vi "datapadding.vi"() -> ()   [LabVIEW 2020]
uses:
  common/record_file_handler/VFH-file_cluster-r140.ctl
  common/record_file_handler/VFH-file_cluster-NanoVNA.ctl
  common/record_file_handler/VFH-VNA_File_Handler.lvlib
panel:
  out "XY Graph":T1(graph)
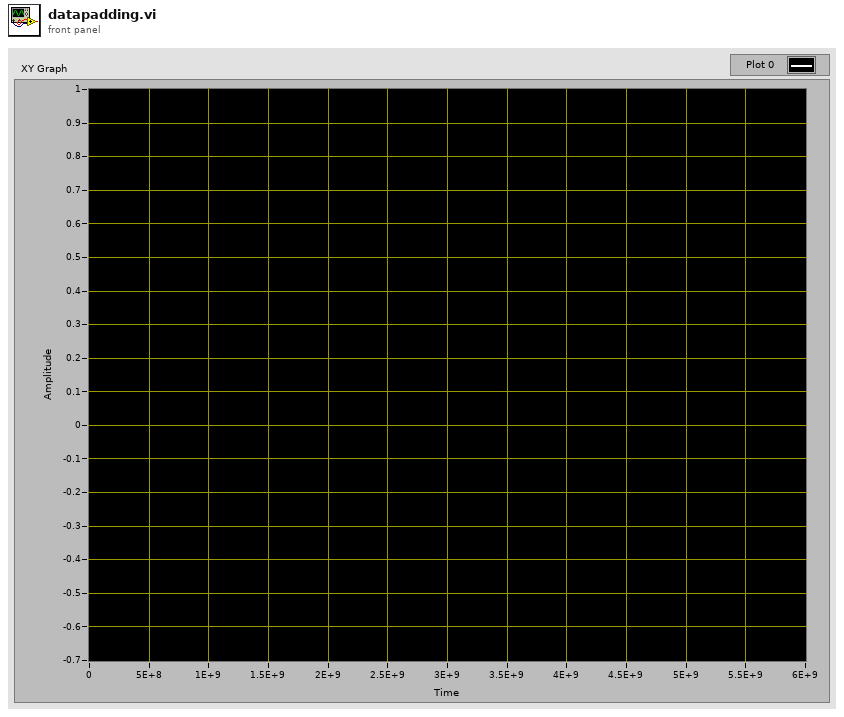
[diagram p1: front panel]
types:
  T1 = cluster{"Frequency":dbl[], "Reflection R":dbl[]}[]
  T2 = typedef "VFH-VNA_File_Handler.lvlib/VFH-file_cluster-NanoVNA.ctl" = cluster{"Frequency":dbl[], "S11_Real":dbl[], "S11_Imag":dbl[], "S21_Real":dbl[], "S21_Imag":dbl[], "S12_Real":dbl[], "S12_Imag":dbl[], "S22_Real":dbl[], "S22_Imag":dbl[]}
  T3 = typedef "VFH-VNA_File_Handler.lvlib/VFH-file_cluster-r140.ctl" = cluster{"Frequency":dbl[], "Permativity'":dbl[], "Permativity''":dbl[], "Q [S/m]":dbl[], "Tan":dbl[], "Reflection R":dbl[], "Reflection I":dbl[]}
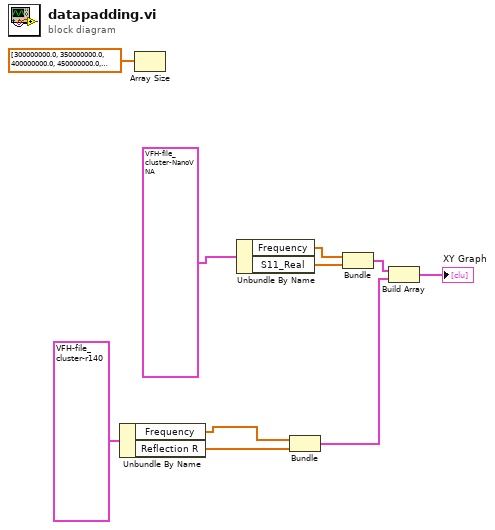
[diagram p0: block diagram]
diagram:
  n1 = Unbundle By Name(T3 {"Frequency"=[300000000.0, 350000000.0, 400000000.0, 450000000.0, 500000000.0, 550000000.0, 600000000.0, 650000000.0, 700000000.0, 750000000.0, 800000000.0, 850000000.0, 900000000.0, 950000000.0, 1000000000.0, 1050000000.0, 1100000000.0, 1150000000.0, 1200000000.0, 1250000000.0, 1300000000.0, 1350000000.0, 1400000000.0, 1450000000.0, 1500000000.0, 1550000000.0, 1600000000.0, 1650000000.0, 1700000000.0, 1750000000.0, 1800000000.0, 1850000000.0, 1900000000.0, 1950000000.0, 2000000000.0, 2050000000.0, 2100000000.0, 2150000000.0, 2200000000.0, 2250000000.0, 2300000000.0, 2350000000.0, 2400000000.0, 2450000000.0, 2500000000.0, 2550000000.0, 2600000000.0, 2650000000.0, 2700000000.0, 2750000000.0, 2800000000.0, 2850000000.0, 2900000000.0, 2950000000.0, 3000000000.0, 3050000000.0, 3100000000.0, 3150000000.0, 3200000000.0, 3250000000.0, 3300000000.0, 3350000000.0, 3400000000.0, 3450000000.0, 3500000000.0, 3550000000.0, 3600000000.0, 3650000000.0, 3700000000.0, 3750000000.0, 3800000000.0, 3850000000.0, 3900000000.0, 3950000000.0, 4000000000.0, 4050000000.0, 4100000000.0, 4150000000.0, 4200000000.0, 4250000000.0, 4300000000.0, 4350000000.0, 4400000000.0, 4450000000.0, 4500000000.0, 4550000000.0, 4600000000.0, 4650000000.0, 4700000000.0, 4750000000.0, 4800000000.0, 4850000000.0, 4900000000.0, 4950000000.0, 5000000000.0, 5050000000.0, 5100000000.0, 5150000000.0, 5200000000.0, 5250000000.0, 5300000000.0, 5350000000.0, 5400000000.0, 5450000000.0, 5500000000.0, 5550000000.0, 5600000000.0, 5650000000.0, 5700000000.0, 5750000000.0, 5800000000.0, 5850000000.0, 5900000000.0, 5950000000.0], "Permativity'"=[79.07108000000001, 79.07034, 79.06462, 79.056, 79.04534, 79.03753999999999, 79.0347, 79.03193999999999, 79.02342, 79.01277999999999, 78.99972, 78.98438, 78.97855999999999, 78.97154, 78.96216, 78.9497, 78.93456, 78.91888, 78.90404, 78.89126000000002, 78.8751, 78.86262, 78.84502, 78.82257999999999, 78.80032000000001, 78.7757, 78.74557999999999, 78.71386, 78.68402, 78.6533, 78.6191, 78.57827999999999, 78.52912, 78.46958, 78.41691999999999, 78.37318, 78.33406, 78.29446, 78.24640000000002, 78.19012000000001, 78.1309, 78.07466, 78.0258, 77.97828, 77.92783999999999, 77.869, 77.80196, 77.72826, 77.64728, 77.56294, 77.47844, 77.39797999999999, 77.31918, 77.24488, 77.17128, 77.09276, 77.01019999999998, 76.92546, 76.83918, 76.75408, 76.67336, 76.59342000000001, 76.51224, 76.42232, 76.33938, 76.2553, 76.16848, 76.07957999999999, 75.9925, 75.90732, 75.82844000000001, 75.75160000000001, 75.67374, 75.59042, 75.50016, 75.40386, 75.33228000000001, 75.23586, 75.12482, 75.01174, 74.90554, 74.8112, 74.72470000000001, 74.64645999999999, 74.56688, 74.5045, 74.42942000000001, 74.3682, 74.296, 74.22968, 74.18003999999999, 74.13322, 74.08314, 74.03887999999999, 73.97104, 73.89056, 73.81594, 73.72461999999999, 73.63058000000001, 73.54686, 73.47466, 73.40158, 73.33064, 73.27372, 73.20532, 73.13356, 73.09074, 73.00046, 72.8972, 72.78979999999999, 72.66766, 72.52906, 72.39554, 72.24091999999999], "Permativity''"=[1.6255039999999998, 1.868498, 2.0571159999999997, 2.2177439999999997, 2.3622919999999996, 2.5154699999999997, 2.6785360000000003, 2.850908, 3.044002, 3.243128, 3.4423440000000007, 3.6347099999999997, 3.8279579999999997, 4.024862000000001, 4.228188, 4.43362, 4.6342099999999995, 4.833124, 5.032642, 5.228612, 5.425520000000001, 5.623486, 5.823044, 6.021953999999999, 6.221154, 6.421606, 6.621852, 6.820505999999999, 7.0202860000000005, 7.221314, 7.42462, 7.6280019999999995, 7.8291319999999995, 8.02201, 8.215602, 8.411694, 8.611638000000001, 8.815472, 9.024792000000001, 9.23303, 9.438149999999998, 9.639506, 9.840016, 10.03886, 10.23822, 10.434259999999998, 10.62636, 10.81722, 11.011700000000001, 11.2103, 11.4122, 11.61576, 11.8175, 12.01362, 12.20212, 12.38604, 12.5691, 12.75498, 12.94442, 13.139000000000001, 13.33632, 13.52916, 13.71348, 13.88894, 14.062120000000002, 14.234300000000001, 14.409719999999998, 14.591159999999999, 14.775060000000002, 14.95574, 15.13636, 15.31298, 15.483160000000002, 15.6504, 15.81628, 15.981440000000001, 16.15642, 16.31804, 16.49034, 16.66446, 16.83074, 16.998400000000004, 17.1663, 17.32796, 17.47976, 17.64352, 17.805699999999998, 17.96982, 18.14518, 18.325300000000002, 18.499299999999998, 18.66046, 18.810859999999998, 18.94634, 19.081899999999997, 19.23704, 19.3982, 19.56258, 19.7285, 19.88428, 20.03192, 20.171139999999998, 20.296879999999998, 20.41714, 20.542180000000002, 20.663259999999998, 20.793979999999998, 20.938679999999998, 21.11282, 21.30238, 21.50122, 21.70846, 21.908160000000002, 22.099800000000005], "Q [S/m]"=[0.0271287, 0.03638146, 0.04577604, 0.05551923999999999, 0.06570876, 0.0769664, 0.08940635999999999, 0.10308999999999999, 0.11853899999999999, 0.1353148, 0.1532018, 0.1718732, 0.19165880000000002, 0.2127132, 0.2352194, 0.2589806, 0.2835878, 0.309204, 0.33596719999999997, 0.3635932, 0.3923774, 0.42233660000000006, 0.453521, 0.4857634, 0.5191366, 0.5537258, 0.589412, 0.6260655999999999, 0.6639314, 0.7030296, 0.7434744, 0.7850581999999999, 0.8275355999999998, 0.8702363999999999, 0.9140898, 0.9593052, 1.0060600000000002, 1.0543980000000002, 1.1045340000000003, 1.155704, 1.20763, 1.260208, 1.313792, 1.3682640000000001, 1.423912, 1.480208, 1.537014, 1.594708, 1.6540120000000003, 1.7150199999999998, 1.7776560000000003, 1.8416700000000001, 1.906532, 1.971584, 2.036464, 2.101606, 2.1676279999999997, 2.235168, 2.3043620000000002, 2.375554, 2.4483279999999996, 2.521362, 2.593852, 2.665678, 2.738024, 2.811148, 2.885876, 2.9628000000000005, 3.0412399999999997, 3.1200300000000003, 3.199818, 3.2797460000000003, 3.359253999999999, 3.439074, 3.5195260000000004, 3.6007279999999993, 3.685092, 3.767344, 3.8529919999999995, 3.94003, 4.026156, 4.113552, 4.201936, 4.289698, 4.375902, 4.465972, 4.556546, 4.648526, 4.744376000000001, 4.842433999999999, 4.9398800000000005, 5.034816, 5.127714, 5.21735, 5.3077559999999995, 5.404424000000001, 5.503655999999999, 5.60471, 5.707116, 5.807495999999999, 5.906328, 6.003494, 6.097367999999999, 6.19029, 6.285334, 6.379862, 6.478058, 6.581386, 6.694846, 6.814214, 6.937613999999999, 7.06486, 7.190802, 7.315175999999999], "Tan"=[0.0205575, 0.02363082, 0.02601812, 0.028052840000000002, 0.029885299999999997, 0.03182628, 0.03389066, 0.03607288, 0.03852024, 0.04104564, 0.04357414, 0.04601808, 0.048468300000000006, 0.05096598, 0.05354698, 0.05615753999999999, 0.058709500000000005, 0.061241659999999996, 0.0637818, 0.06627618, 0.0687862, 0.07130736, 0.07385428000000001, 0.0763989, 0.07894833999999999, 0.08151758, 0.08409177999999999, 0.08664936, 0.08922122, 0.09181196, 0.09443788, 0.0970752, 0.0996972, 0.1022308, 0.1047682, 0.1073288, 0.10993499999999998, 0.1125936, 0.11533820000000002, 0.1180844, 0.12079899999999999, 0.12346539999999999, 0.12611219999999998, 0.128739, 0.13138060000000001, 0.133998, 0.1365824, 0.13916699999999999, 0.1418172, 0.144532, 0.147295, 0.1500784, 0.1528406, 0.1555264, 0.15811780000000003, 0.16066419999999998, 0.1632134, 0.1658096, 0.168461, 0.17118319999999998, 0.17393679999999997, 0.1766362, 0.179232, 0.18173940000000002, 0.184205, 0.1866662, 0.1891822, 0.19178820000000002, 0.1944278, 0.19702619999999998, 0.1996136, 0.20214720000000003, 0.2046036, 0.2070418, 0.20948700000000003, 0.21194459999999998, 0.2144688, 0.21689180000000002, 0.2195058, 0.222158, 0.22469260000000002, 0.2272174, 0.2297276, 0.2321338, 0.2344172, 0.2368118, 0.23922919999999998, 0.24163259999999998, 0.24422859999999996, 0.24687260000000003, 0.2493842, 0.25171520000000003, 0.2539152, 0.25589699999999993, 0.25796420000000003, 0.26034520000000005, 0.2627916, 0.2653468, 0.267939, 0.27036239999999995, 0.272637, 0.2748058, 0.27678579999999997, 0.2786422, 0.2806106, 0.2825414, 0.2844954, 0.2868298, 0.2896246, 0.2926564, 0.2958842, 0.29930660000000003, 0.3026174, 0.3059182], "Reflection R"=[0.9563704, 0.9414002, 0.9247411999999999, 0.9059240000000001, 0.8855024, 0.8633542000000001, 0.8395902, 0.8143844000000001, 0.7883522000000001, 0.7609335999999999, 0.7324565999999999, 0.7032166000000001, 0.6739214, 0.6433788, 0.6123486, 0.5807945999999999, 0.5489086, 0.5175911999999999, 0.48633800000000005, 0.4556078, 0.4245774, 0.3932044, 0.3617632, 0.3310108, 0.30149380000000003, 0.2725546, 0.24442719999999998, 0.2156358, 0.18743959999999998, 0.1598338, 0.1335008, 0.1081772, 0.08306316, 0.05885234, 0.03523574, 0.01166094, -0.0112239, -0.03295492, -0.05388126, -0.07428524, -0.094318, -0.11344019999999999, -0.13217859999999998, -0.150481, -0.16820279999999999, -0.1856306, -0.20200420000000002, -0.21786219999999998, -0.23093919999999998, -0.2456136, -0.26064980000000004, -0.2747486, -0.288448, -0.3011898, -0.3128512, -0.324151, -0.3351994, -0.34643159999999995, -0.3575456, -0.36866319999999997, -0.3791824, -0.38919739999999997, -0.39882399999999996, -0.4075296, -0.41552039999999996, -0.42310299999999995, -0.43109340000000007, -0.43894420000000006, -0.4473358, -0.45564020000000005, -0.4632442, -0.4704846, -0.4770398, -0.4829552, -0.48858379999999996, -0.4945457999999999, -0.5007142, -0.5070786, -0.5129922, -0.5186019999999999, -0.5234748, -0.528023, -0.5318077999999999, -0.5361992000000001, -0.5410092000000001, -0.5462636000000001, -0.5514082, -0.5562567999999999, -0.5603596, -0.5636416, -0.5665338, -0.5734653999999999, -0.5766823999999999, -0.5790569999999999, -0.582066, -0.5858825999999999, -0.5894844, -0.5926942, -0.5958612000000001, -0.598381, -0.6025852, -0.6041282, -0.6085657999999999, -0.6097562, -0.6116034000000001, -0.614562, -0.6169844, -0.6190056, -0.6235666, -0.6252584, -0.6264618000000001, -0.6298440000000001, -0.630876, -0.6311298], "Reflection I"=[-0.2724698, -0.31527580000000005, -0.3569708, -0.39736259999999995, -0.43687820000000005, -0.47402820000000007, -0.5103186, -0.5448104, -0.577333, -0.6084758000000001, -0.6379132000000001, -0.6652576, -0.6909622000000001, -0.7150329999999999, -0.7374517999999999, -0.7579908, -0.7767417999999999, -0.7933899999999999, -0.8087218, -0.8230147999999999, -0.8356515999999999, -0.8470384, -0.8573310000000001, -0.8647012000000001, -0.8711336, -0.8764986, -0.8819204, -0.8860628, -0.8892678, -0.8904706000000001, -0.8907684, -0.8908866, -0.8899744, -0.8882756, -0.8864772000000001, -0.8838202000000001, -0.880477, -0.8765978000000001, -0.8724959999999999, -0.8680396, -0.8626924, -0.8571676, -0.8515086000000001, -0.8456258, -0.8394454, -0.8324263999999999, -0.8253484, -0.8182224, -0.8124207999999999, -0.8055906, -0.7983317999999999, -0.790975, -0.7835146, -0.7760478, -0.7686808, -0.7610172000000001, -0.7532197999999999, -0.745435, -0.7377613999999999, -0.7300576, -0.722393, -0.715164, -0.7083980000000001, -0.701418, -0.6942134, -0.686626, -0.6787333999999999, -0.6708944000000001, -0.6632136000000001, -0.6562418, -0.6494382, -0.6427252, -0.6360187999999999, -0.6294966, -0.6226278, -0.6150616000000001, -0.6078354, -0.6010314, -0.5946328000000001, -0.5886338, -0.582608, -0.5765022, -0.5701457999999999, -0.563566, -0.557402, -0.550292, -0.5437841999999999, -0.5379995999999999, -0.5325564, -0.5275712, -0.5224264, -0.5134958000000001, -0.5091794000000001, -0.5030577999999999, -0.49717399999999995, -0.4918436, -0.4859821999999999, -0.4802664, -0.4752636, -0.47164339999999993, -0.4649464, -0.46106559999999996, -0.4557778, -0.45077480000000003, -0.445472, -0.4396398, -0.4347174, -0.4301863999999999, -0.4259030000000001, -0.42265040000000004, -0.4174022, -0.411794, -0.40744800000000003, -0.40280940000000004]} ("Handled data")) -> ("Frequency"=w8:dbl[], "Reflection R"=w7:dbl[])
  n2 = Array Size(array=dbl[] [300000000.0, 350000000.0, 400000000.0, 450000000.0, 500000000.0, 550000000.0, 600000000.0, 650000000.0, 700000000.0, 750000000.0, 800000000.0, 850000000.0, 900000000.0, 950000000.0, 1000000000.0, 1050000000.0, 1100000000.0, 1150000000.0, 1200000000.0, 1250000000.0, 1300000000.0, 1350000000.0, 1400000000.0, 1450000000.0, 1500000000.0, 1550000000.0, 1600000000.0, 1650000000.0, 1700000000.0, 1750000000.0, 1800000000.0, 1850000000.0, 1900000000.0, 1950000000.0, 2000000000.0, 2050000000.0, 2100000000.0, 2150000000.0, 2200000000.0, 2250000000.0, 2300000000.0, 2350000000.0, 2400000000.0, 2450000000.0, 2500000000.0, 2550000000.0, 2600000000.0, 2650000000.0, 2700000000.0, 2750000000.0, 2800000000.0, 2850000000.0, 2900000000.0, 2950000000.0, 3000000000.0, 3050000000.0, 3100000000.0, 3150000000.0, 3200000000.0, 3250000000.0, 3300000000.0, 3350000000.0, 3400000000.0, 3450000000.0, 3500000000.0, 3550000000.0, 3600000000.0, 3650000000.0, 3700000000.0, 3750000000.0, 3800000000.0, 3850000000.0, 3900000000.0, 3950000000.0, 4000000000.0, 4050000000.0, 4100000000.0, 4150000000.0, 4200000000.0, 4250000000.0, 4300000000.0, 4350000000.0, 4400000000.0, 4450000000.0, 4500000000.0, 4550000000.0, 4600000000.0, 4650000000.0, 4700000000.0, 4750000000.0, 4800000000.0, 4850000000.0, 4900000000.0, 4950000000.0, 5000000000.0, 5050000000.0, 5100000000.0, 5150000000.0, 5200000000.0, 5250000000.0, 5300000000.0, 5350000000.0, 5400000000.0, 5450000000.0, 5500000000.0, 5550000000.0, 5600000000.0, 5650000000.0, 5700000000.0, 5750000000.0, 5800000000.0, 5850000000.0, 5900000000.0, 5950000000.0] ("Waveform Graph")) -> ()  [unwired: 1 out]
  n3 = Unbundle By Name(T2 {"Frequency"=array[801 elements], "S11_Real"=array[801 elements], "S11_Imag"=array[801 elements], "S21_Real"=array[801 elements], "S21_Imag"=array[801 elements], "S12_Real"=array[801 elements], "S12_Imag"=array[801 elements], "S22_Real"=array[801 elements], "S22_Imag"=array[801 elements]} ("avg output")) -> ("Frequency"=w5:dbl[], "S11_Real"=w4:dbl[])
  n4 = Bundle("Frequency"=w8, "Reflection R"=w7) -> (w2:cluster{"Frequency":dbl[], "Reflection R":dbl[]})  [unwired: 1 in]
  n5 = Bundle("Frequency"=w5, "S11_Real"=w4) -> (w3:cluster{"Frequency":dbl[], "S11_Real":dbl[]})  [unwired: 1 in]
  n6 = Build Array(w3, w2) -> (→"XY Graph":T1)
